vi "NumericCaseStructure.vi"() -> ()   [LabVIEW 2018]
panel:
  in  "?":bool
  out "Out of Range":bool
  out "7 - 10":bool
  out "4 - 6":bool
  out "0 - 3":bool
  in  "Numeric":dbl
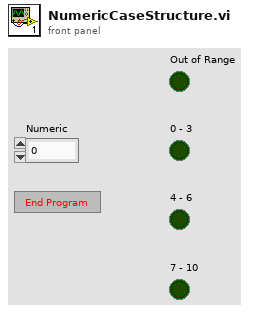
[diagram p1: front panel]
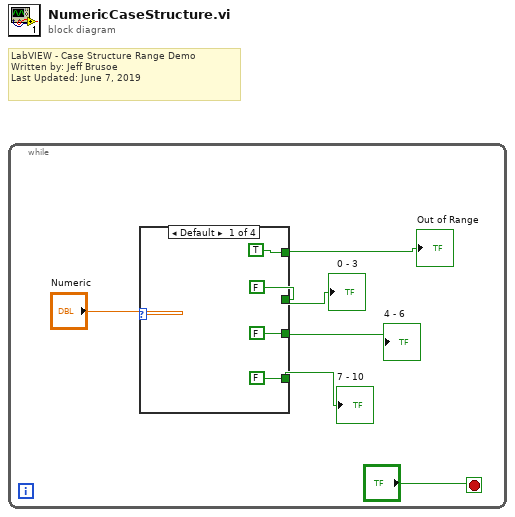
[diagram p0: block diagram]
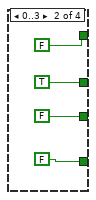
[diagram p2: hidden frame]
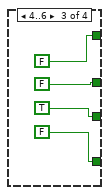
[diagram p3: hidden frame]
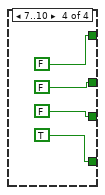
[diagram p4: hidden frame]
diagram:
  # "LabVIEW - Case Structure Range Demo\nWritten by: Jeff Brusoe\nLast Updated: June 7, 2019"
  n1 = while {
    stop <- "?" stop-if-true
    n2 = case shown="Default" "Numeric" {
      tunnel: [FALSE FALSE FALSE TRUE] -> w6
      tunnel: [FALSE FALSE TRUE FALSE] -> w5
      tunnel: [FALSE TRUE FALSE FALSE] -> w4
      tunnel: [TRUE FALSE FALSE FALSE] -> w2
      frame Default {
      }
      frame 0..3 {
      }
      frame 4..6 {
      }
      frame 7..10 {
      }
    }
    "0 - 3" <- w4
    "4 - 6" <- w5
    "7 - 10" <- w6
    "Out of Range" <- w2
  }
